vi "AutomatedBeamGage_ManualStepTable.vi"() -> ()   [LabVIEW 2018]
uses:
  C:/Program Files/Spiricon/BeamSquared/M2.Automation.dll
  M2.Automation.dll
panel:
  out "RunStatus":i32(ring) items=["READY", "RUNNING", "RUN_FINISHED", "UNAVAILABLE", "ABORTED", "LOADING", "ERROR"]
  in  "Save Run Settings":bool
  in  "Shutdown Server":bool
  in  "ManualStepArray":dbl[](array[numeric])
  in  "Save Step Table":bool
  in  "Start/Stop Run":bool
  out "FrameAnalyzerStatus":i32
  in  "Model":string
  in  "Comment":string
  in  "CorrectForSmear":bool
  in  "FittedDivergence":bool
  in  "LaserLocation":dbl
  in  "FocalLength":dbl
  in  "WaveLength":dbl
  in  "SerialNumber":string
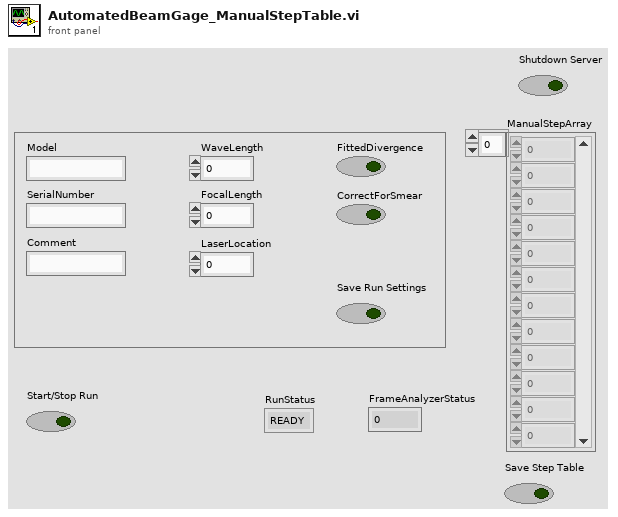
[diagram p1: front panel]
types:
  T1 = cluster{"notifier out":refnum<notifier>, "new reference":refnum<k24>}
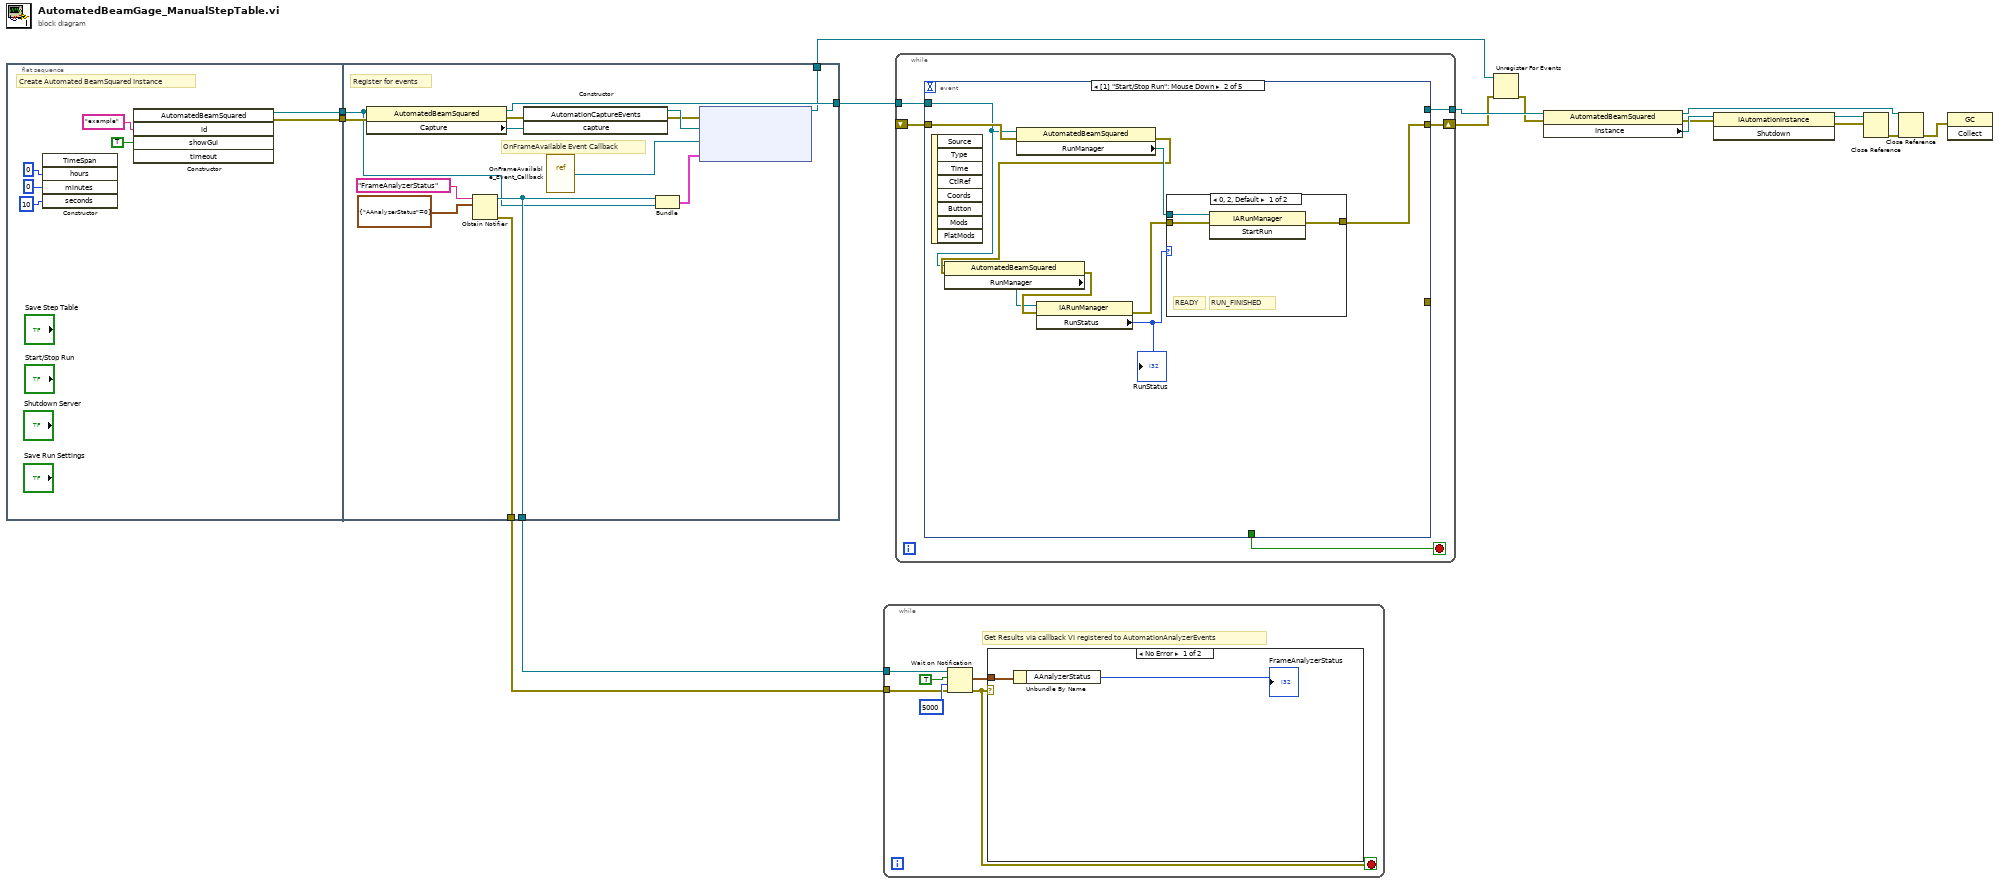
[diagram p0: block diagram]
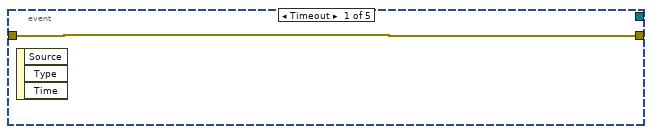
[diagram p3: hidden frame]
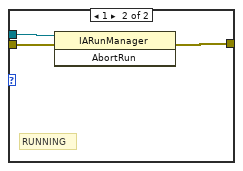
[diagram p4: hidden frame]
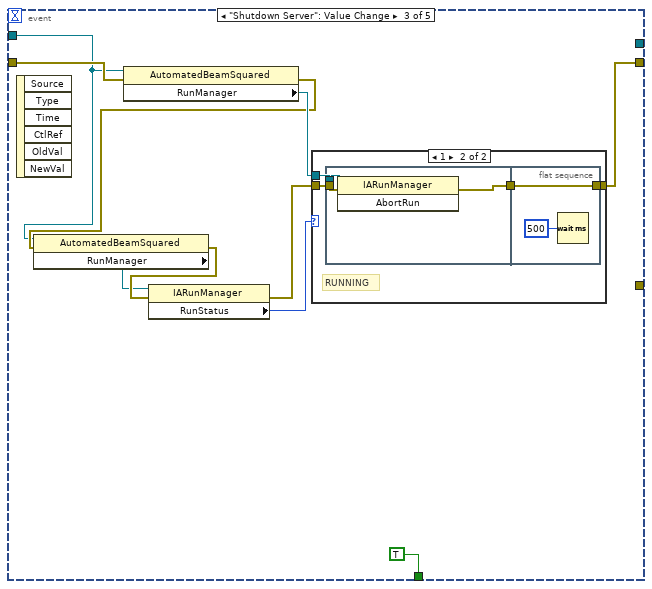
[diagram p5: hidden frame]
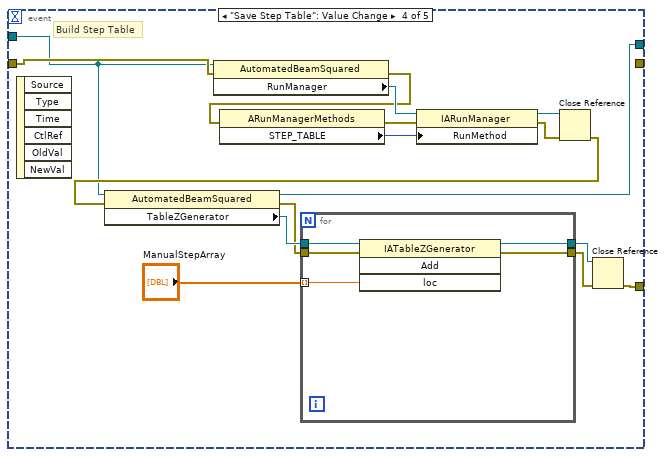
[diagram p7: hidden frame]
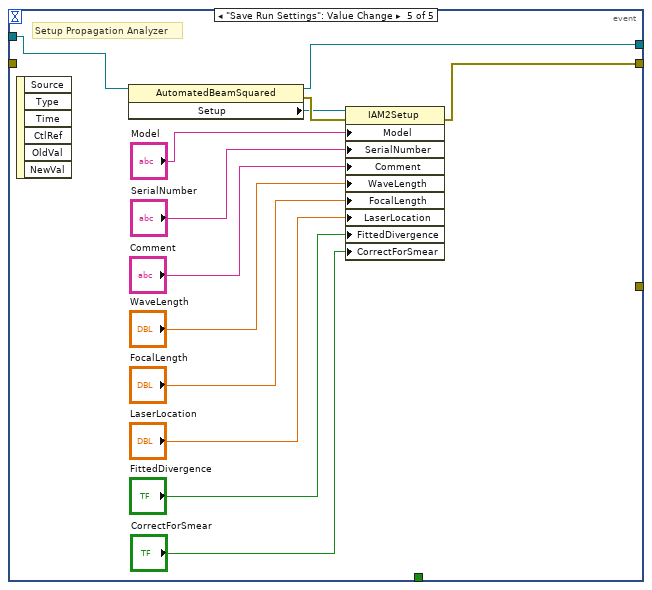
[diagram p8: hidden frame]
diagram:
  n1 = flat-sequence {
    tunnel: [w18] -> w16
    tunnel: [w17] -> w15
    tunnel: [w28] -> w8
    tunnel: w15 -> [w25]
    tunnel: w16 -> [w31]
    tunnel: [w27] -> w2
    tunnel: [w26] -> w6
    tunnel: [w24] -> w1
    frame #0 {
      # "Create Automated BeamSquared Instance"
      n2 = constructor class="TimeSpan"("hours"=0, "minutes"=0, "seconds"=10) -> ()  [unwired: 3 in, 6 out]
      n3 = constructor class="AutomatedBeamSquared"("id"="example", "showGui"=TRUE) -> (reference out=w17:refnum<k24>, error out=w18:errorcluster)  [unwired: 4 in, 4 out]
    }
    frame #1 {
      # "OnFrameAvailable Event Callback"
      # "Register for events"
      n4 = property class="AutomatedBeamSquared"(reference=w25, error in=w31) -> (reference out=w26:refnum<k24>, error out=w30:errorcluster, "Capture"=w32:refnum<k24>)
      n5 = Obtain Notifier(name (unnamed)="FrameAnalyzerStatus", notification data type=cluster{"AAnalyzerStatus":i32} {"AAnalyzerStatus"=0}) -> (notifier out=w27:refnum<notifier>, error out=w28:errorcluster)  [unwired: 2 in, 1 out]
      n6 = constructor class="AutomationCaptureEvents"(error in=w30, "capture"=w32) -> (reference out=w37:refnum<k24>, error out=w36:errorcluster)  [unwired: 2 in, 2 out]
      n7 = vi-ref "OnFrameAvailable_Event_Callback.vi"() -> ("vi reference"=w34:refnum<vi>)
      n8 = Bundle("notifier out"=w27, "new reference"=w25) -> (w29:T1)  [unwired: 1 in]
      n9 = node(w36, w37, w34, w29) -> (w24:refnum<k27>)  [unwired: 1 in, 1 out]
    }
  }
  n10 = while {
    tunnel: w8 -> [w41]
    tunnel: w2 -> [w38]
    stop <- w39 stop-if-true
    # "Get Results via callback VI registered to AutomationAnalyzerEvents"
    n11 = Wait on Notification(notifier=w38, ignore previous (F)=TRUE, timeout in ms (-1)=5000, error in (no error)=w41) -> (notification=w40:cluster{"AAnalyzerStatus":i32}, error out=w39:errorcluster)  [unwired: 2 out]
    n12 = case shown="No Error" w39 {
      tunnel: w40 -> [w45 _]
      frame No Error {
        n13 = Unbundle By Name(w45) -> ("AAnalyzerStatus"=→"FrameAnalyzerStatus":i32)
      }
      frame Error {
      }
    }
  }
  n14 = while {
    shift-right: [w49] -> w4
    shift-left: _ -> [w50]
    tunnel: [w47] -> w7
    tunnel: w6 -> [w46]
    stop <- w48 stop-if-true
    n15 = event shown="[1] \"Start/Stop Run\": Mouse Down" {
      selector: _ -> [_ _ _ _ _]
      dyn-events: _ -> [_ _ _ _ _]
      timeout: _ -> [_ _ _ _ _]
      tunnel: w50 -> [w51 w60 w76 w92 _]
      tunnel: [w51 w53 w69 _ w108] -> w49
      tunnel: [_ _ TRUE _ _] -> w48
      tunnel: [_ _ _ w99 _] -> _
      tunnel: [_ _ _ w88 w109] -> w47
      tunnel: w46 -> [_ w52 w67 w87 w110]
      event Timeout {
        n16 = event-data() -> ()  [unwired: 1 in, 3 out]
      }
      event "Start/Stop Run": Mouse Down {
        n17 = event-data() -> ()  [unwired: 1 in, 8 out]
        n18 = property class="AutomatedBeamSquared"(reference=w52, error in=w60) -> (error out=w57:errorcluster, "RunManager"=w59:refnum<k24>)  [unwired: 1 out]
        n19 = property class="AutomatedBeamSquared"(reference=w52, error in=w57) -> (error out=w58:errorcluster, "RunManager"=w56:refnum<k24>)  [unwired: 1 out]
        n20 = property class="IARunManager"(reference=w56, error in=w58) -> (error out=w54:errorcluster, "RunStatus"=w55:i32)  [unwired: 1 out]
        "RunStatus" <- w55
        n21 = case shown="0, 2, Default" w55 {
          tunnel: w59 -> [w63 w66]
          tunnel: w54 -> [w62 w65]
          tunnel: [w61 w64] -> w53
          frame 0, 2, Default {
            # "RUN_FINISHED"
            # "READY"
            n22 = invoke class="IARunManager" method="StartRun"(reference=w63, error in=w62) -> (error out=w61:errorcluster)  [unwired: 1 in, 2 out]
          }
          frame 1 {
            # "RUNNING"
            n23 = invoke class="IARunManager" method="AbortRun"(reference=w66, error in=w65) -> (error out=w64:errorcluster)  [unwired: 1 in, 2 out]
          }
        }
      }
      event "Shutdown Server": Value Change {
        n24 = event-data() -> ()  [unwired: 1 in, 6 out]
        n25 = property class="AutomatedBeamSquared"(reference=w67, error in=w76) -> (error out=w73:errorcluster, "RunManager"=w75:refnum<k24>)  [unwired: 1 out]
        n26 = property class="AutomatedBeamSquared"(reference=w67, error in=w73) -> (error out=w74:errorcluster, "RunManager"=w72:refnum<k24>)  [unwired: 1 out]
        n27 = property class="IARunManager"(reference=w72, error in=w74) -> (error out=w70:errorcluster, "RunStatus"=w71:i32)  [unwired: 1 out]
        n28 = case shown="1" w71 {
          tunnel: w75 -> [_ w81]
          tunnel: w70 -> [w77 w80]
          tunnel: [w77 w79] -> w69
          frame 0, 2, Default {
            # "RUN_FINISHED"
            # "READY"
          }
          frame 1 {
            # "RUNNING"
            n29 = flat-sequence {
              tunnel: w81 -> [w84]
              tunnel: w80 -> [w83]
              tunnel: [w82] -> w78
              tunnel: [w86] -> w79
              tunnel: w78 -> [w86]
              frame #0 {
                n30 = invoke class="IARunManager" method="AbortRun"(reference=w84, error in=w83) -> (error out=w82:errorcluster)  [unwired: 1 in, 2 out]
              }
              frame #1 {
                n31 = Wait (ms)(milliseconds to wait=u32 500) -> ()  [unwired: 1 out]
              }
            }
          }
        }
      }
      event "Save Step Table": Value Change {
        # "Build Step Table"
        n32 = event-data() -> ()  [unwired: 1 in, 6 out]
        n33 = property class="AutomatedBeamSquared"(reference=w87, error in=w92) -> (error out=w94:errorcluster, "RunManager"=w96:refnum<k24>)  [unwired: 1 out]
        n34 = property class="ARunManagerMethods"(error in=w94) -> (error out=w95:errorcluster, "STEP_TABLE"=w93:i32)  [unwired: 1 in, 1 out]
        n35 = property class="IARunManager"(reference=w96, error in=w95, "RunMethod"=w93) -> (reference out=w97:refnum<k24>, error out=w98:errorcluster)
        n36 = Close Reference(reference=w97, error in (no error)=w98) -> (error out=w89:errorcluster)
        n37 = property class="AutomatedBeamSquared"(reference=w87, error in=w89) -> (reference out=w88:refnum<k24>, error out=w101:errorcluster, "TableZGenerator"=w102:refnum<k24>)
        n38 = for {
          tunnel: "ManualStepArray" -> [w107] mode=indexing
          tunnel: w101 -> [w106]
          tunnel: [w105] -> w91
          tunnel: [w104] -> w90
          tunnel: w102 -> [w103]
          n39 = invoke class="IATableZGenerator" method="Add"(reference=w103, error in=w106, "loc"=w107) -> (reference out=w104:refnum<k24>, error out=w105:errorcluster)  [unwired: 1 in, 2 out]
        }
        n40 = Close Reference(reference=w90, error in (no error)=w91) -> (error out=w99:errorcluster)
      }
      event "Save Run Settings": Value Change {
        # "Setup Propagation Analyzer"
        n41 = event-data() -> ()  [unwired: 1 in, 6 out]
        n42 = property class="AutomatedBeamSquared"(reference=w110) -> (reference out=w109:refnum<k24>, error out=w112:errorcluster, "Setup"=w111:refnum<k24>)  [unwired: 1 in]
        n43 = property class="IAM2Setup"(reference=w111, error in=w112, "Model"="Model", "SerialNumber"="SerialNumber", "Comment"="Comment", "WaveLength"="WaveLength", "FocalLength"="FocalLength", "LaserLocation"="LaserLocation", "FittedDivergence"="FittedDivergence", "CorrectForSmear"="CorrectForSmear") -> (error out=w108:errorcluster)  [unwired: 1 out]
      }
    }
  }
  n44 = Unregister For Events(event registration refnum=w1, error in=w4) -> (error out=w3:errorcluster)
  n45 = property class="AutomatedBeamSquared"(reference=w7, error in=w3) -> (reference out=w11:refnum<k24>, error out=w9:errorcluster, "Instance"=w10:refnum<k24>)
  n46 = invoke class="IAutomationInstance" method="Shutdown"(reference=w10, error in=w9) -> (reference out=w12:refnum<k24>, error out=w13:errorcluster)  [unwired: 1 in, 1 out]
  n47 = Close Reference(reference=w12, error in (no error)=w13) -> (error out=w14:errorcluster)
  n48 = Close Reference(reference=w11, error in (no error)=w14) -> (error out=w5:errorcluster)
  n49 = invoke class="GC" method="Collect"(error in=w5) -> ()  [unwired: 2 in, 3 out]
